vi "To JSON.vi"(5 "enable LabVIEW extensions? (T)":bool=TRUE, 6 "Pretty Print?":bool, 7 "LVClass Serializer":refnum<class "JSONtext LVClass Serializer.lvclass">, 8 "error in (no error)":errorcluster, 11 "Mock JSON Serializable in":refnum<class "Mock JSON Serializable.lvclass">) -> (0 "error out":errorcluster, 2 "<JSON>":string, 3 "Mock JSON Serializable out":refnum<class "Mock JSON Serializable.lvclass">)   [LabVIEW 2017, in "JSON Serializable Serializer Tests.lvlib" / "Mock JSON Serializable.lvclass"]
doc: "Creates a JSON string from an object."
uses:
  Mock JSON Serializable.lvclass
  <vilib>/JDP Science/JSONtext/LVClass Serializer/JSONtext LVClass Serializer.lvclass
  Mock JSON Serializable.lvclass/Mock JSON Serializable.ctl
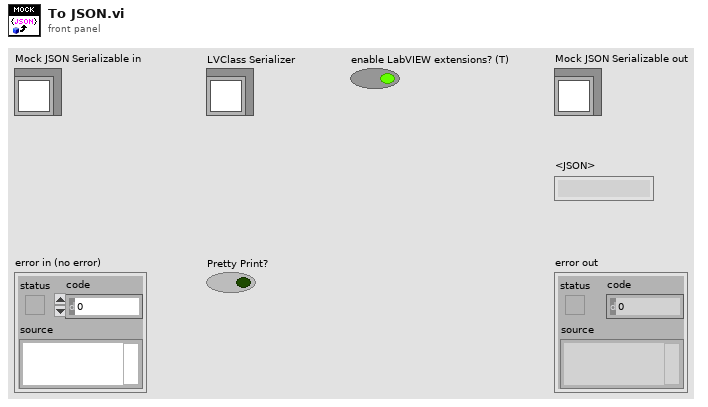
[diagram p1: front panel]
types:
  T1 = cluster{"LVClass Serializer":refnum<class "JSONtext LVClass Serializer.lvclass">, "enable LabVIEW extensions? (T)":bool, "Pretty Print?":bool, "error in (no error)":errorcluster}
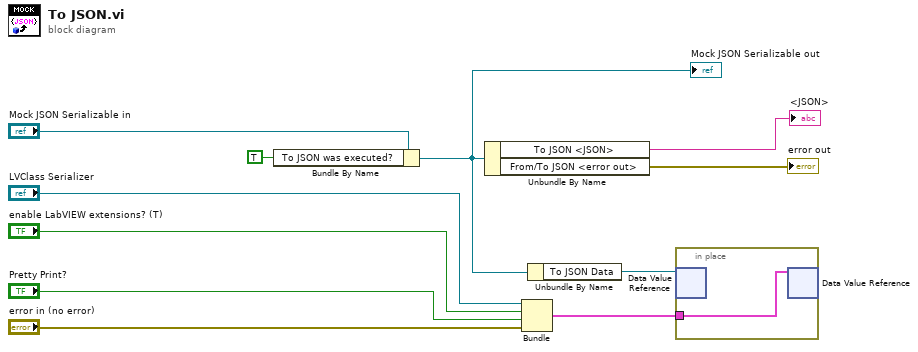
[diagram p0: block diagram]
diagram:
  n1 = Bundle By Name(cluster="Mock JSON Serializable in", "To JSON was executed?"=TRUE) -> (w2:refnum<class "Mock JSON Serializable.lvclass">)
  "Mock JSON Serializable out" <- w2
  n2 = Unbundle By Name(w2) -> ("To JSON <JSON>"=→"<JSON>":string, "From/To JSON <error out>"=→"error out":errorcluster)
  n3 = Bundle("LVClass Serializer"="LVClass Serializer", "enable LabVIEW extensions? (T)"="enable LabVIEW extensions? (T)", "Pretty Print?"="Pretty Print?", "error in (no error)"="error in (no error)") -> (w6:T1)  [unwired: 1 in]
  n4 = Unbundle By Name(w2) -> ("To JSON Data"=w7:refnum<data-value>)
  n5 = in-place {
    in-place-border: w6 -> [w12]
    n6 = in-place-dvr #1(w7) -> ()  [unwired: 2 out]
    n7 = in-place-dvr #1(w12) -> ()  [unwired: 2 out]
  }
